vi "MiniBatchKMeans.vi"(8 "error in":errorcluster) -> (0 "error out":errorcluster, 3 "out":refnum<class "MiniBatchKMeans.lvclass">)   [LabVIEW 2020]
doc: "Mini-Batch K-Means clustering.\n\n Read more in the :ref:`User Guide <mini_batch_kmeans>`.\n\n Parameters\n ----------\n\n n_clusters : int, default=8\n The number of clusters to form as well as the number of\n centroids to generate.\n\n init : {'k-means++', 'random'}, callable or array-like of shape (n_clusters, n_features), default='k-means++'\n Method for initialization:\n\n 'k-means++' : selects initial cluster centers for k-mean\n clustering in a smart way to speed up convergence. See section\n Notes in k_init for more details.\n\n 'random': choose `n_clusters` observations (rows) at random from data\n for the initial centroids.\n\n If an array is passed, it should be of shape (n_clusters, n_features)\n and gives the initial centers.\n\n If a callable is passed, it should take arguments X, n_clusters and a\n random state and return an initialization.\n\n max_iter : int, default=100\n Maximum number of iterations over the complete dataset before\n stopping independently of any early stopping criterion heuristics.\n\n batch_size : int, default=100\n Size of the mini batches.\n\n verbose : int, default=0\n Verbosity mode.\n\n compute_labels : bool, default=True\n Compute label assignment and inertia for the complete dataset\n once the minibatch optimization has converged in fit.\n\n random_state : int, RandomState instance or None, default=None\n Determines random number generation for centroid initialization and\n random reassignment. Use an int to make the randomness deterministic.\n See :term:`Glossary <random_state>`.\n\n tol : float, default=0.0\n Control early stopping based on the relative center changes as\n measured by a smoothed, variance-normalized of the mean center\n squared position changes. This early stopping heuristics is\n closer to the one used for the batch variant of the algorithms\n but induces a slight computational and memory overhead over the\n inertia heuristic.\n\n To disable convergence detection based on normalized center\n change, set tol to 0.0 (default).\n\n max_no_improvement : int, default=10\n Control early stopping based on the consecutive number of mini\n batches that does not yield an improvement on the smoothed inertia.\n\n To disable convergence detection based on inertia, set\n max_no_improvement to None.\n\n init_size : int, default=None\n Number of samples to randomly sample for speeding up the\n initialization (sometimes at the expense of accuracy): the\n only algorithm is initialized by running a batch KMeans on a\n random subset of the data. This needs to be larger than n_clusters.\n\n If `None`, `init_size= 3 * batch_size`.\n\n n_init : int, default=3\n Number of random initializations that are tried.\n In contrast to KMeans, the algorithm is only run once, using the\n best of the ``n_init`` initializations as measured by inertia.\n\n reassignment_ratio : float, default=0.01\n Control the fraction of the maximum number of counts for a\n center to be reassigned. A higher value means that low count\n centers are more easily reassigned, which means that the\n model will take longer to converge, but should converge in a\n better clustering.\n\n Attributes\n ----------\n\n cluster_centers_ : ndarray of shape (n_clusters, n_features)\n Coordinates of cluster centers.\n\n labels_ : int\n Labels of each point (if compute_labels is set to True).\n\n inertia_ : float\n The value of the inertia criterion associated with the chosen\n partition (if compute_labels is set to True). The inertia is\n defined as the sum of square distances of samples to their nearest\n neighbor.\n\n n_iter_ : int\n Number of batches processed.\n\n counts_ : ndarray of shape (n_clusters,)\n Weigth sum of each cluster.\n\n .. deprecated:: 0.24\n This attribute is deprecated in 0.24 and will be removed in\n 1.1 (renaming of 0.26).\n\n init_size_ : int\n The effective number of samples used for the initialization.\n\n .. deprecated:: 0.24\n This attribute is deprecated in 0.24 and will be removed in\n 1.1 (renaming of 0.26).\n\n See Also\n --------\n KMeans : The classic implementation of the clustering method based on the\n Lloyd's algorithm. It consumes the whole set of input data at each\n iteration.\n\n Notes\n -----\n See https://www.eecs.tufts.edu/~dsculley/papers/fastkmeans.pdf\n\n \nAvailable methods:\nGet Attributes\nGet Params\nSet Params"
uses:
  MiniBatchKMeans.lvclass
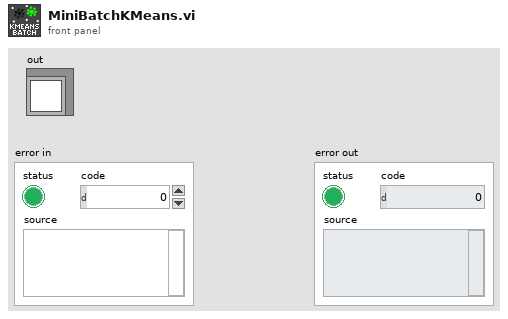
[diagram p1: front panel]
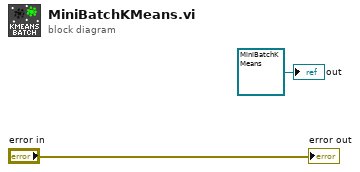
[diagram p0: block diagram]
diagram:
  "out" <- refnum<class "MiniBatchKMeans.lvclass"> refnum ("model")
  "error out" <- "error in"
